vi "Connect.vi"(0 "Communication":T1(ring), 5 "Terminator":enum32{"rdiCr", "rdiLf", "rdiCrLf"}(ring), 7 "Address/Device number":string, 9 "Port":i32, 11 "error in (no error)":errorcluster, 12 "GPIBBoard":i32) -> (4 "Reference out":refnum<k24>, 15 "error out":errorcluster)   [LabVIEW 2017]
uses:
  C:/Users/Ssantec_Test/Documents/Instrument_DLL_Sample_Labview_20220902_Ver1.2.2/DLL/x86/InstrumentDLL.dll
  DLL/x86/InstrumentDLL.dll
panel:
  # "input"
  # "output"
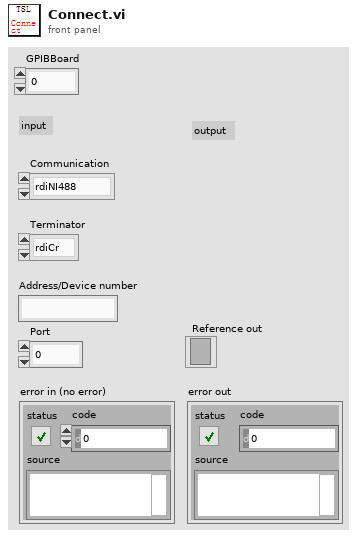
[diagram p1: front panel]
types:
  T1 = enum32{"rdiNI488", "rdiNIvisa", "rdikysightvisa", "rdiUSB", "rdiLAN"}
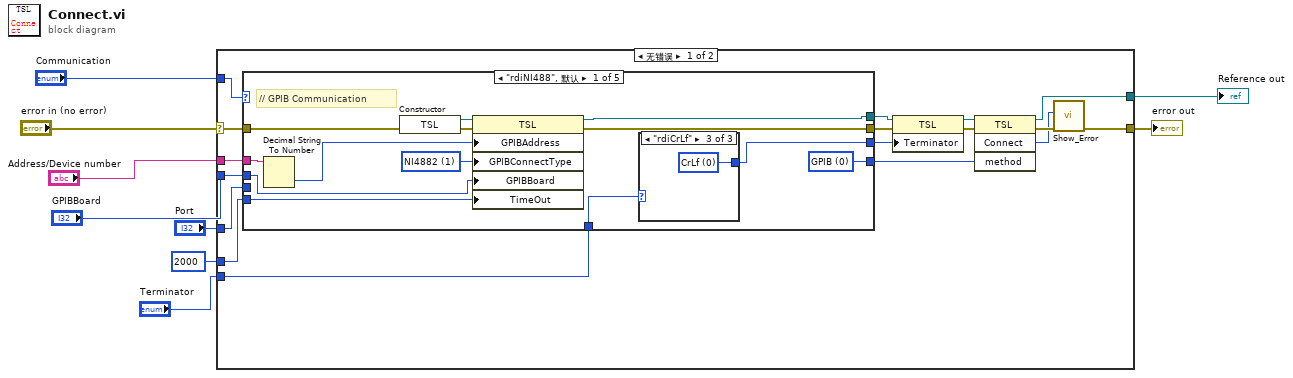
[diagram p0: block diagram]
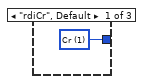
[diagram p2: hidden frame]
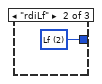
[diagram p3: hidden frame]
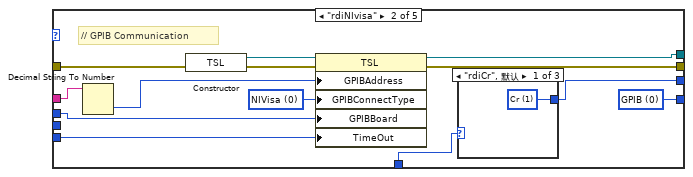
[diagram p4: hidden frame]
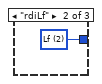
[diagram p5: hidden frame]
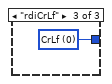
[diagram p6: hidden frame]
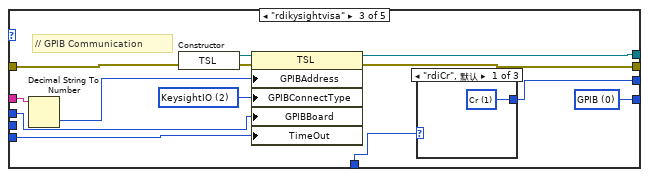
[diagram p7: hidden frame]
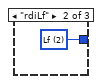
[diagram p8: hidden frame]
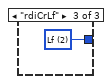
[diagram p9: hidden frame]
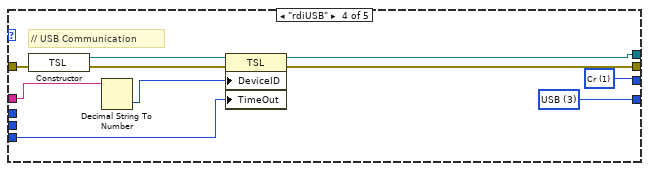
[diagram p10: hidden frame]
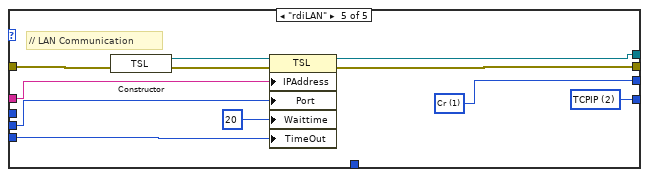
[diagram p11: hidden frame]
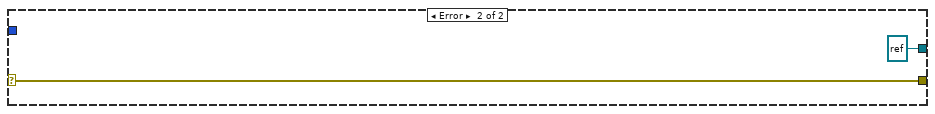
[diagram p12: hidden frame]
diagram:
  n1 = case shown="无错误" "error in (no error)" {
    selector: "error in (no error)" -> [w16 w96]
    tunnel: "Address/Device number" -> [w26 _]
    tunnel: "Communication" -> [w25 _]
    tunnel: "Port" -> [w24 _]
    tunnel: 2000 ("TimeOut") -> [w23 _]
    tunnel: "GPIBBoard" -> [w21 _]
    tunnel: [w20 refnum<k24> refnum ("new reference")] -> w5
    tunnel: [w17 w96] -> w4
    tunnel: "Terminator" -> [w11 _]
    frame No Error {
      n2 = case shown="\"rdiNI488\", 默认" w25 {
        tunnel: w26 -> [w39 w55 w71 w77 w95]
        tunnel: w24 -> [_ _ _ _ w93]
        tunnel: w23 -> [w38 w54 w70 w83 w92]
        tunnel: [w37 w51 w67 w80 w88] -> w15
        tunnel: [w36 w52 w68 w81 w89] -> w14
        tunnel: [w35 w53 w69 w82 w90] -> w22
        tunnel: w21 -> [w34 w49 w65 _ _]
        tunnel: w16 -> [w33 w48 w64 w78 w87]
        tunnel: w11 -> [w28 w44 w60 _ _]
        tunnel: [w27 w43 w59 w75 w85] -> w10
        frame "rdiNI488", Default {
          w31 = 1 items=["NIVisa", "NI4882", "KeysightIO"] ("GPIBConnectType 2")
          w35 = 0 items=["GPIB", "C232C", "TCPIP", "USB"] ("method 2")
          # "// GPIB Communication"
          n3 = Decimal String To Number(string=w39) -> (number=w32:i32)  [unwired: 2 in, 1 out]
          n4 = constructor class="TSL"(error in=w33) -> (reference out=w30:refnum<k24>, error out=w29:errorcluster)  [unwired: 2 in, 1 out]
          n5 = property class="TSL"(reference=w30, error in=w29, "GPIBAddress"=w32, "GPIBConnectType"=w31, "GPIBBoard"=w34, "TimeOut"=w38) -> (reference out=w37:refnum<k24>, error out=w36:errorcluster)
          n6 = case shown="\"rdiCrLf\"" w28 {
            tunnel: [w40 w41 w42] -> w27
            frame "rdiCr", Default {
              w40 = 1 items=["CrLf", "Cr", "Lf"] ("Terminator")
            }
            frame "rdiLf" {
              w41 = 2 items=["CrLf", "Cr", "Lf"] ("Terminator")
            }
            frame "rdiCrLf" {
              w42 = 0 items=["CrLf", "Cr", "Lf"] ("Terminator")
            }
          }
        }
        frame "rdiNIvisa" {
          w50 = 0 items=["NIVisa", "NI4882", "KeysightIO"] ("GPIBConnectType 2")
          w53 = 0 items=["GPIB", "C232C", "TCPIP", "USB"] ("method 2")
          # "// GPIB Communication"
          n7 = Decimal String To Number(string=w55) -> (number=w47:i32)  [unwired: 2 in, 1 out]
          n8 = constructor class="TSL"(error in=w48) -> (reference out=w46:refnum<k24>, error out=w45:errorcluster)  [unwired: 2 in, 1 out]
          n9 = property class="TSL"(reference=w46, error in=w45, "GPIBAddress"=w47, "GPIBConnectType"=w50, "GPIBBoard"=w49, "TimeOut"=w54) -> (reference out=w51:refnum<k24>, error out=w52:errorcluster)
          n10 = case shown="\"rdiCr\", 默认" w44 {
            tunnel: [w56 w57 w58] -> w43
            frame "rdiCr", Default {
              w56 = 1 items=["CrLf", "Cr", "Lf"] ("Terminator")
            }
            frame "rdiLf" {
              w57 = 2 items=["CrLf", "Cr", "Lf"] ("Terminator")
            }
            frame "rdiCrLf" {
              w58 = 0 items=["CrLf", "Cr", "Lf"] ("Terminator")
            }
          }
        }
        frame "rdikysightvisa" {
          w66 = 2 items=["NIVisa", "NI4882", "KeysightIO"] ("GPIBConnectType 2")
          w69 = 0 items=["GPIB", "C232C", "TCPIP", "USB"] ("method 2")
          # "// GPIB Communication"
          n11 = Decimal String To Number(string=w71) -> (number=w63:i32)  [unwired: 2 in, 1 out]
          n12 = constructor class="TSL"(error in=w64) -> (reference out=w62:refnum<k24>, error out=w61:errorcluster)  [unwired: 2 in, 1 out]
          n13 = property class="TSL"(reference=w62, error in=w61, "GPIBAddress"=w63, "GPIBConnectType"=w66, "GPIBBoard"=w65, "TimeOut"=w70) -> (reference out=w67:refnum<k24>, error out=w68:errorcluster)
          n14 = case shown="\"rdiCr\", 默认" w60 {
            tunnel: [w72 w73 w74] -> w59
            frame "rdiCr", Default {
              w72 = 1 items=["CrLf", "Cr", "Lf"] ("Terminator")
            }
            frame "rdiLf" {
              w73 = 2 items=["CrLf", "Cr", "Lf"] ("Terminator")
            }
            frame "rdiCrLf" {
              w74 = 2 items=["CrLf", "Cr", "Lf"] ("Terminator")
            }
          }
        }
        frame "rdiUSB" {
          w75 = 1 items=["CrLf", "Cr", "Lf"] ("Terminator")
          w82 = 3 items=["GPIB", "C232C", "TCPIP", "USB"] ("method")
          # "// USB Communication"
          n15 = constructor class="TSL"(error in=w78) -> (reference out=w84:refnum<k24>, error out=w79:errorcluster)  [unwired: 2 in, 1 out]
          n16 = Decimal String To Number(string=w77) -> (number=w76:i32)  [unwired: 2 in, 1 out]
          n17 = property class="TSL"(reference=w84, error in=w79, "DeviceID"=w76, "TimeOut"=w83) -> (reference out=w80:refnum<k24>, error out=w81:errorcluster)
        }
        frame "rdiLAN" {
          w85 = 1 items=["CrLf", "Cr", "Lf"] ("Terminator")
          w90 = 2 items=["GPIB", "C232C", "TCPIP", "USB"] ("method")
          # "// LAN Communication"
          n18 = constructor class="TSL"(error in=w87) -> (reference out=w94:refnum<k24>, error out=w86:errorcluster)  [unwired: 2 in, 1 out]
          n19 = property class="TSL"(reference=w94, error in=w86, "IPAddress"=w95, "Port"=w93, "Waittime"=20, "TimeOut"=w92) -> (reference out=w88:refnum<k24>, error out=w89:errorcluster)
        }
      }
      n20 = property class="TSL"(reference=w15, error in=w14, "Terminator"=w10) -> (reference out=w12:refnum<k24>, error out=w13:errorcluster)
      n21 = invoke on="调用节点" class="TSL" method="Connect"(reference=w12, error in=w13, "method"=w22) -> (reference out=w20:refnum<k24>, error out=w19:errorcluster, "Connect"=w18:i32)  [unwired: 1 in, 1 out]
      n22 = call "Show_Error.vi"("error in (no error)"=w19, "Error"=w18) -> ("error out"=w17:errorcluster)  [unwired: 9 in]
    }
    frame Error {
    }
  }
  "Reference out" <- w5
  "error out" <- w4
